vi "acquireVI.vi"(8 "error in (no error)":errorcluster, 9 "Enum":T1, 10 "Param in":T2, 11 "Queue in":refnum<queue>) -> (0 "error out":errorcluster, 3 "Queue out":refnum<queue>)   [LabVIEW 2023]
uses:
  Param out.ctl
  enum_read.ctl
  enum_FGV.ctl
  <vilib>/DAQmx/read.llb/DAQmx Read (Analog 1D Wfm NChan NSamp).vi
  <vilib>/DAQmx/create/channels.llb/DAQmx Create Channel (AI-Acceleration-Accelerometer).vi
  <vilib>/DAQmx/create/channels.llb/DAQmx Create Channel (AI-Voltage-Basic).vi
  <vilib>/DAQmx/configure/timing.llb/DAQmx Timing (Sample Clock).vi
  <vilib>/DAQmx/miscellaneous.llb/DAQmx Fill In Error Info.vi
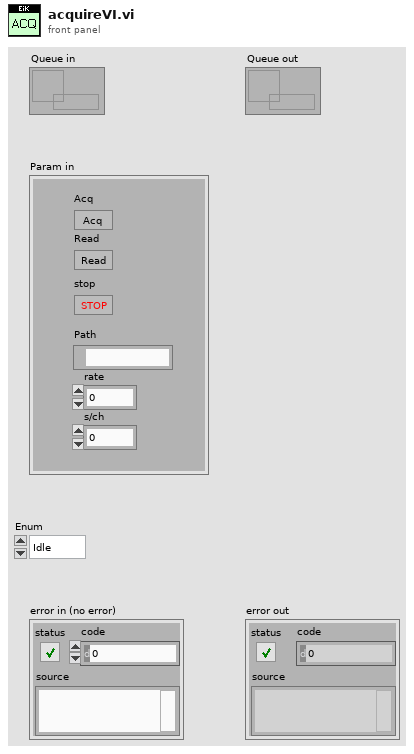
[diagram p1: front panel]
types:
  T1 = typedef "enum_read.ctl" = enum16{"Idle", "Init", "Read", "End"}
  T2 = typedef "Param out.ctl" = cluster{"Acq":bool, "stop":bool, "Path":path, "rate":dbl, "s/ch":dbl, "Read":bool}
  T3 = typedef "enum_FGV.ctl" = enum16{"Get", "Set"}
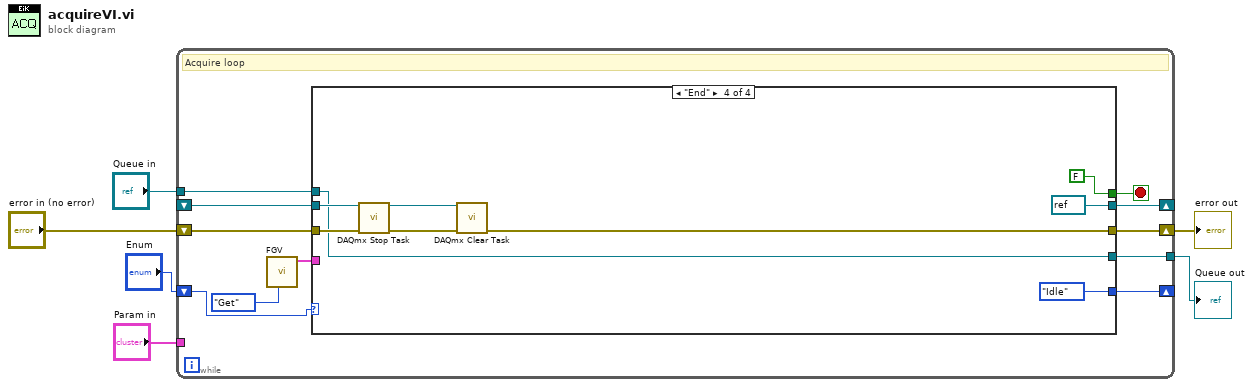
[diagram p0: block diagram]
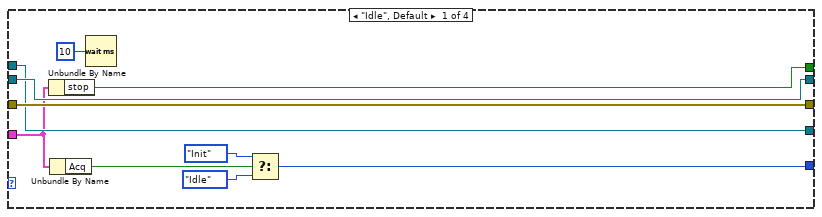
[diagram p2: hidden frame]
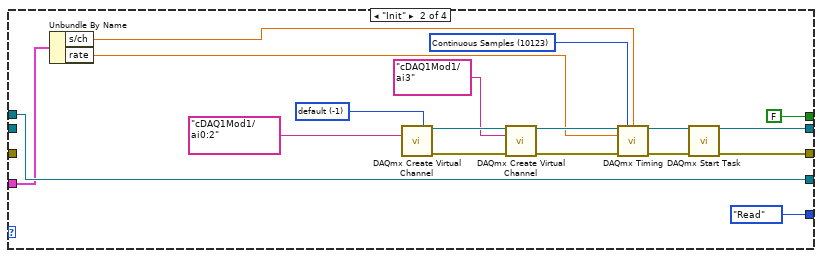
[diagram p3: hidden frame]
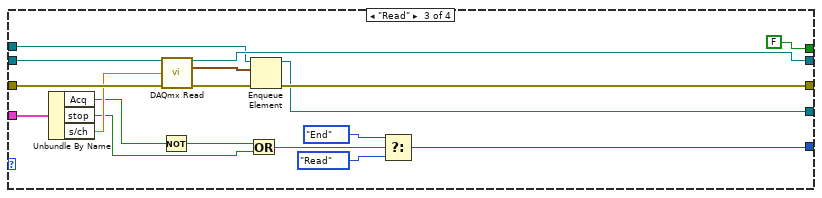
[diagram p4: hidden frame]
diagram:
  n1 = while {
    shift-right: [w16] -> _
    shift-left: "Enum" -> [w17]
    shift-right: [w14] -> w3
    shift-left: "error in (no error)" -> [w12]
    shift-right: [w15] -> _
    shift-left: _ -> [w13]
    tunnel: "Queue in" -> [w11]
    tunnel: [w10] -> w2
    tunnel: "Param in" -> [_]
    stop <- w7 stop-if-true
    # "Acquire loop"
    n2 = call "FGV.vi"("Action"=enum_FGV."Get") -> ("Param out"=w9:T2)  [unwired: 10 in]
    n3 = case shown="\"End\"" w17 {
      tunnel: [w26 enum_read."Read" w60 enum_read."Idle"] -> w16
      tunnel: [w24 w41 w56 w68] -> w14
      tunnel: [w25 w40 w61 refnum<k21> refnum ("task out")] -> w15
      tunnel: w13 -> [w25 _ w63 w70]
      tunnel: w12 -> [w24 _ w62 w69]
      tunnel: w11 -> [w21 w32 w55 w65]
      tunnel: [w21 w32 w54 w65] -> w10
      tunnel: w9 -> [w18 w31 w52 _]
      tunnel: [w19 FALSE ("stop") FALSE ("stop") FALSE ("stop")] -> w7
      frame "Idle", Default {
        n4 = Unbundle By Name(w18) -> ("stop"=w19:bool)
        n5 = Unbundle By Name(w18) -> ("Acq"=w20:bool)
        n6 = Wait (ms)(milliseconds to wait=u32 10) -> ()  [unwired: 1 out]
        n7 = Select(t=enum_read."Init", s=w20, f=enum_read."Idle") -> (s? t:f=w26:T1)
      }
      frame "Init" {
        w42 = -1 items=["default"=-1, "RSE"=10083, "NRSE"=10078, "Differential"=10106, "Pseudodifferential"=12529] ("input terminal configuration")
        w43 = 10123 items=["Finite Samples"=10178, "Continuous Samples"=10123, "Hardware Timed Single Point"=12522] ("sample mode")
        n8 = Unbundle By Name(w31) -> ("s/ch"=w29:dbl, "rate"=w30:dbl)
        n9 = call-poly <vilib>:"DAQmx Create Virtual Channel.vi"("input terminal configuration"=w42, "physical channels"=tag "cDAQ1Mod1/ai0:2") -> ("task out"=w37:refnum<k21>, "error out"=w35:errorcluster)  [unwired: 12 in]
        n10 = call-poly <vilib>:"DAQmx Create Virtual Channel.vi"("task in"=w37, "physical channels"=tag "cDAQ1Mod1/ai3", "error in"=w35) -> ("task out"=w36:refnum<k21>, "error out"=w34:errorcluster)  [unwired: 11 in]
        n11 = call-poly <vilib>:"DAQmx Timing.vi"("task/channels in"=w36, "sample mode"=w43, "samples per channel"=w29, "rate"=w30, "error in"=w34) -> ("task out"=w45:refnum<k21>, "error out"=w44:errorcluster)  [unwired: 9 in]
        n12 = call <vilib>:"DAQmx Start Task.vi"("task/channels in"=w45, "error in"=w44) -> ("task out"=w40:refnum<k21>, "error out"=w41:errorcluster)  [unwired: 12 in]
      }
      frame "Read" {
        n13 = Unbundle By Name(w52) -> ("Acq"=w47:bool, "stop"=w48:bool, "s/ch"=w51:dbl)
        n14 = Not(x=w47) -> (.not. x?=w46:bool)
        n15 = call-poly <vilib>:"DAQmx Read.vi"("task/channels in"=w63, "number of samples per channel"=w51, "error in"=w62) -> ("task out"=w61:refnum<k21>, "data"=w53:waveform(dbl)[], "error out"=w57:errorcluster)  [unwired: 10 in]
        n16 = Or(x=w46, y=w48) -> (x .or. y?=w50:bool)
        n17 = Enqueue Element(queue=w55, element=w53, error in (no error)=w57) -> (queue out=w54:refnum<queue>, error out=w56:errorcluster)  [unwired: 1 in, 1 out]
        n18 = Select(t=enum_read."End", s=w50, f=enum_read."Read") -> (s? t:f=w60:T1)
      }
      frame "End" {
        n19 = call <vilib>:"DAQmx Stop Task.vi"("task/channels in"=w70, "error in"=w69) -> ("task out"=w72:refnum<k21>, "error out"=w71:errorcluster)  [unwired: 12 in]
        n20 = call <vilib>:"DAQmx Clear Task.vi"("task in"=w72, "error in"=w71) -> ("error out"=w68:errorcluster)  [unwired: 13 in]
      }
    }
  }
  "error out" <- w3
  "Queue out" <- w2
